vi "unflattenAccelerationFromXML_Array.vi"(8 "error in (no error)":errorcluster, 9 "accelerationUnitInXML":T1, 10 "xmlString":string, 11 "accelerationForType":dbl[unit][](array[numeric])=[0.2617993877991494, 0.5235987755982988, 0.7853981633974482, 1.0471975511965976]) -> (0 "error out":errorcluster, 3 "acceleration":dbl[unit][](array[numeric]))   [LabVIEW 2016, in "UnitsAndXML.lvlib"]
uses:
  <userlib>/Common/UnitsAndXML/UnitsAndXML.lvlib
  <userlib>/Common/UnitsAndXML/FlattenItemWithUnitToXML/FlattenAccelerationToXML/AccelerationUnit.ctl
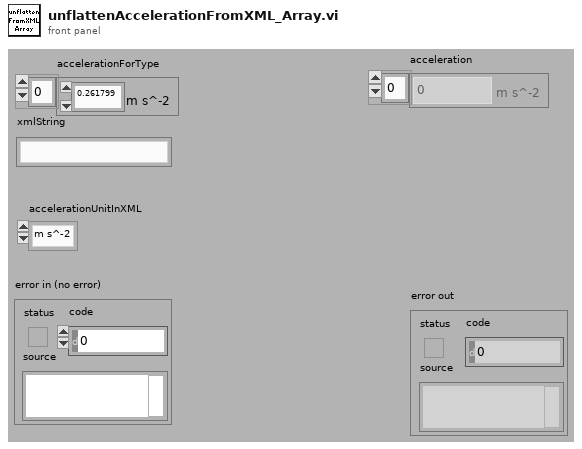
[diagram p1: front panel]
types:
  T1 = typedef "UnitsAndXML.lvlib/AccelerationUnit.ctl" = enum16{"m s^-2"}
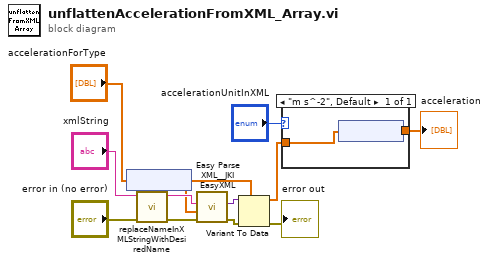
[diagram p0: block diagram]
diagram:
  n1 = node("accelerationForType") -> (w8:dbl[])
  n2 = call <userlib>:"replaceNameInXMLStringWithDesiredName.vi"("error in"="error in (no error)", "xmlString"="xmlString") -> ("error out"=w1:errorcluster, "revisedXMLString"=w9:string)  [unwired: 8 in]
  n3 = call <vilib>:"Easy Parse XML__JKI EasyXML.vi"("error in (no error)"=w1, "LabVIEW Data (Type)"=w8, "XML String"=w9) -> ("error out"=w4:errorcluster, "LabVIEW Data"=w11:variant)  [unwired: 7 in]
  n4 = Variant To Data(error in=w4, type=w8, Variant=w11) -> (data=w7:dbl[], error out=→"error out":errorcluster)
  n5 = case shown="\"m s^-2\", Default" "accelerationUnitInXML" {
    tunnel: w7 -> [w13]
    tunnel: [w14] -> w6
    frame "m s^-2", Default {
      n6 = node(w13) -> (w14:dbl[unit][])
    }
  }
  "acceleration" <- w6
